vi "获取公式.vi"(10 "量程选择":enum16{"低量程", "高量程", "0-2量程"}(ring), 11 "测量模式(公式)":u16(ring)=1 items=["水样测试"=1, "标样核查"=2, "零点核查"=3, "跨度核查"=4, "空白测试"=5, "平行样"=6, "加标回收"=7]) -> (3 "方程系数":cluster{"K":dbl, "b":dbl, "X^2":dbl} {"X^2" format="%#.6g"; "b" format="%#.6g"; "K" format="%#.6g"})   [LabVIEW 2016, in "斯坦道CODMn.lvlib"]
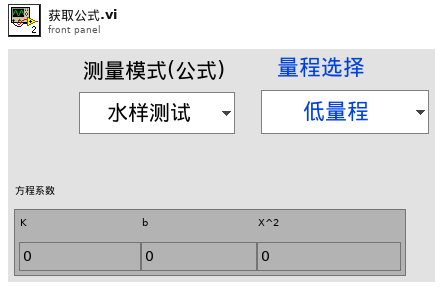
[diagram p1: front panel]
types:
  T1 = cluster{"数组 2[0]":sgl, "数组 2[1]":sgl, "数组 2[2]":sgl, "数组 2[3]":sgl, "数组 2[4]":sgl, "数组 2[5]":sgl, "数组 2[6]":sgl, "数组 2[7]":sgl, "数组 2[8]":sgl, "数组 2[9]":sgl, "数组 2[10]":sgl, "数组 2[11]":sgl, "数组 2[12]":sgl, "数组 2[13]":sgl, "数组 2[14]":sgl, "数组 2[15]":sgl, "数组 2[16]":sgl, "数组 2[17]":sgl, "数组 2[18]":sgl, "数组 2[19]":sgl, "数组 2[20]":sgl, "数组 2[21]":sgl, "数组 2[22]":sgl, "数组 2[23]":sgl, "数组 2[24]":sgl, "数组 2[25]":sgl, "数组 2[26]":sgl, "数组 2[27]":sgl, "数组 2[28]":sgl, "数组 2[29]":sgl, "数组 2[30]":sgl, "数组 2[31]":sgl, "数组 2[32]":sgl, "数组 2[33]":sgl, "数组 2[34]":sgl, "数组 2[35]":sgl, "数组 2[36]":sgl, "数组 2[37]":sgl, "数组 2[38]":sgl, "数组 2[39]":sgl, "数组 2[40]":sgl, "数组 2[41]":sgl}
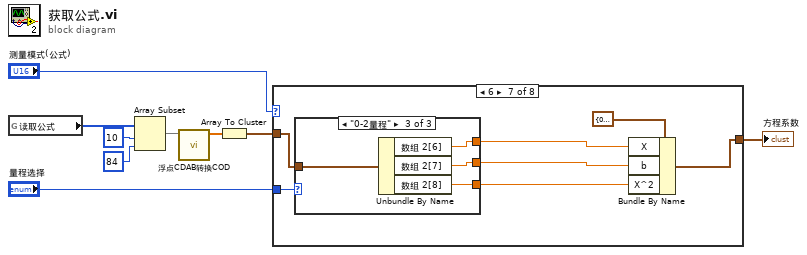
[diagram p0: block diagram]
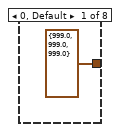
[diagram p2: hidden frame]
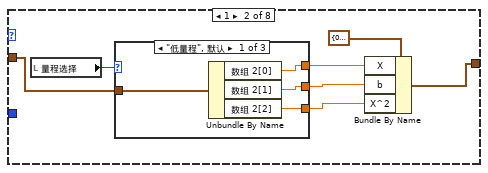
[diagram p3: hidden frame]
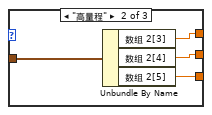
[diagram p4: hidden frame]
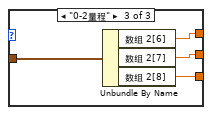
[diagram p5: hidden frame]
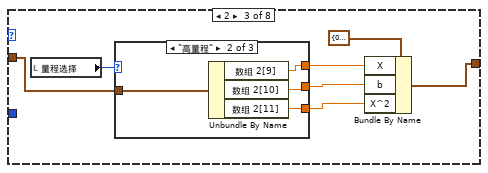
[diagram p6: hidden frame]
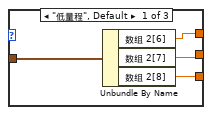
[diagram p7: hidden frame]
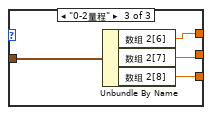
[diagram p8: hidden frame]
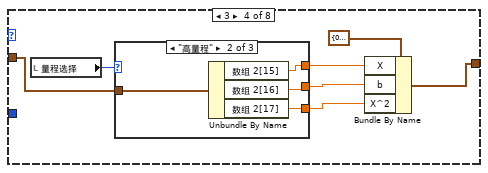
[diagram p9: hidden frame]
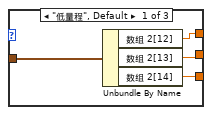
[diagram p10: hidden frame]
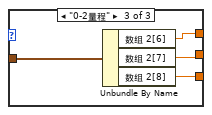
[diagram p11: hidden frame]
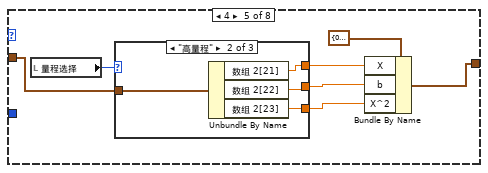
[diagram p12: hidden frame]
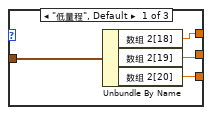
[diagram p13: hidden frame]
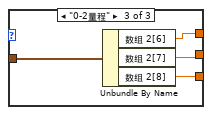
[diagram p14: hidden frame]
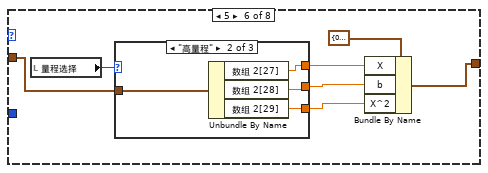
[diagram p15: hidden frame]
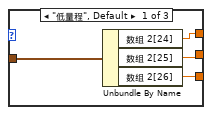
[diagram p16: hidden frame]
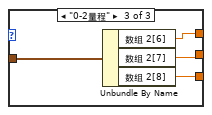
[diagram p17: hidden frame]
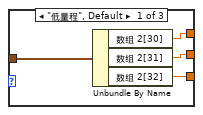
[diagram p18: hidden frame]
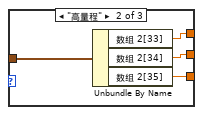
[diagram p19: hidden frame]
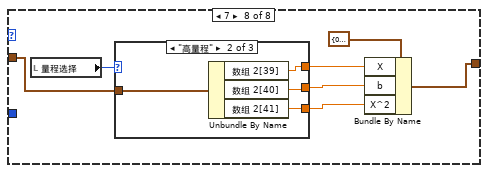
[diagram p20: hidden frame]
diagram:
  n1 = global read "COD内部交互全局.vi" "读取公式"() -> (w9:u16[])
  n2 = Array Subset(array=w9, index=10 ("索引"), length=84 ("长度")) -> (w6:u16[])
  n3 = call "浮点CDAB转换COD.vi"("数组"=w6) -> ("数组 2"=w7:sgl[])  [unwired: 10 in]
  n4 = Array To Cluster(array=w7) -> (cluster=w8:T1)
  n5 = case shown="6" "测量模式(公式)" {
    tunnel: [cluster{"X":dbl, "b":dbl, "X^2":dbl} {"X"=999.0, "b"=999.0, "X^2"=999.0} ("方程系数") w12 w31 w50 w69 w88 w108 w126] -> w1
    tunnel: w8 -> [_ w11 w30 w49 w68 w87 w107 w125]
    tunnel: "量程选择" -> [_ _ _ _ _ _ w106 _]
    frame 0, Default {
    }
    frame 1 {
      n6 = local read "量程选择"() -> (w14:enum16{"低量程", "高量程", "0-2量程"})
      n7 = case shown="\"低量程\", 默认" w14 {
        tunnel: w11 -> [w21 w25 w29]
        tunnel: [w20 w24 w28] -> w17
        tunnel: [w19 w23 w27] -> w16
        tunnel: [w18 w22 w26] -> w15
        frame "低量程", Default {
          n8 = Unbundle By Name(w21) -> ("数组 2[0]"=w20:sgl, "数组 2[1]"=w19:sgl, "数组 2[2]"=w18:sgl)
        }
        frame "高量程" {
          n9 = Unbundle By Name(w25) -> ("数组 2[3]"=w24:sgl, "数组 2[4]"=w23:sgl, "数组 2[5]"=w22:sgl)
        }
        frame "0-2量程" {
          n10 = Unbundle By Name(w29) -> ("数组 2[6]"=w28:sgl, "数组 2[7]"=w27:sgl, "数组 2[8]"=w26:sgl)
        }
      }
      n11 = Bundle By Name(cluster=cluster{"X":dbl, "b":dbl, "X^2":dbl} {"X"=0.0, "b"=0.0, "X^2"=0.0} ("方程系数"), "X"=w17, "b"=w16, "X^2"=w15) -> (w12:cluster{"X":dbl, "b":dbl, "X^2":dbl})
    }
    frame 2 {
      n12 = local read "量程选择"() -> (w33:enum16{"低量程", "高量程", "0-2量程"})
      n13 = case shown="\"高量程\"" w33 {
        tunnel: w30 -> [w40 w44 w48]
        tunnel: [w39 w43 w47] -> w36
        tunnel: [w38 w42 w46] -> w35
        tunnel: [w37 w41 w45] -> w34
        frame "低量程", Default {
          n14 = Unbundle By Name(w40) -> ("数组 2[6]"=w39:sgl, "数组 2[7]"=w38:sgl, "数组 2[8]"=w37:sgl)
        }
        frame "高量程" {
          n15 = Unbundle By Name(w44) -> ("数组 2[9]"=w43:sgl, "数组 2[10]"=w42:sgl, "数组 2[11]"=w41:sgl)
        }
        frame "0-2量程" {
          n16 = Unbundle By Name(w48) -> ("数组 2[6]"=w47:sgl, "数组 2[7]"=w46:sgl, "数组 2[8]"=w45:sgl)
        }
      }
      n17 = Bundle By Name(cluster=cluster{"X":dbl, "b":dbl, "X^2":dbl} {"X"=0.0, "b"=0.0, "X^2"=0.0} ("方程系数"), "X"=w36, "b"=w35, "X^2"=w34) -> (w31:cluster{"X":dbl, "b":dbl, "X^2":dbl})
    }
    frame 3 {
      n18 = local read "量程选择"() -> (w52:enum16{"低量程", "高量程", "0-2量程"})
      n19 = case shown="\"高量程\"" w52 {
        tunnel: w49 -> [w59 w63 w67]
        tunnel: [w58 w62 w66] -> w55
        tunnel: [w57 w61 w65] -> w54
        tunnel: [w56 w60 w64] -> w53
        frame "低量程", Default {
          n20 = Unbundle By Name(w59) -> ("数组 2[12]"=w58:sgl, "数组 2[13]"=w57:sgl, "数组 2[14]"=w56:sgl)
        }
        frame "高量程" {
          n21 = Unbundle By Name(w63) -> ("数组 2[15]"=w62:sgl, "数组 2[16]"=w61:sgl, "数组 2[17]"=w60:sgl)
        }
        frame "0-2量程" {
          n22 = Unbundle By Name(w67) -> ("数组 2[6]"=w66:sgl, "数组 2[7]"=w65:sgl, "数组 2[8]"=w64:sgl)
        }
      }
      n23 = Bundle By Name(cluster=cluster{"X":dbl, "b":dbl, "X^2":dbl} {"X"=0.0, "b"=0.0, "X^2"=0.0} ("方程系数"), "X"=w55, "b"=w54, "X^2"=w53) -> (w50:cluster{"X":dbl, "b":dbl, "X^2":dbl})
    }
    frame 4 {
      n24 = local read "量程选择"() -> (w71:enum16{"低量程", "高量程", "0-2量程"})
      n25 = case shown="\"高量程\"" w71 {
        tunnel: w68 -> [w78 w82 w86]
        tunnel: [w77 w81 w85] -> w74
        tunnel: [w76 w80 w84] -> w73
        tunnel: [w75 w79 w83] -> w72
        frame "低量程", Default {
          n26 = Unbundle By Name(w78) -> ("数组 2[18]"=w77:sgl, "数组 2[19]"=w76:sgl, "数组 2[20]"=w75:sgl)
        }
        frame "高量程" {
          n27 = Unbundle By Name(w82) -> ("数组 2[21]"=w81:sgl, "数组 2[22]"=w80:sgl, "数组 2[23]"=w79:sgl)
        }
        frame "0-2量程" {
          n28 = Unbundle By Name(w86) -> ("数组 2[6]"=w85:sgl, "数组 2[7]"=w84:sgl, "数组 2[8]"=w83:sgl)
        }
      }
      n29 = Bundle By Name(cluster=cluster{"X":dbl, "b":dbl, "X^2":dbl} {"X"=0.0, "b"=0.0, "X^2"=0.0} ("方程系数"), "X"=w74, "b"=w73, "X^2"=w72) -> (w69:cluster{"X":dbl, "b":dbl, "X^2":dbl})
    }
    frame 5 {
      n30 = local read "量程选择"() -> (w90:enum16{"低量程", "高量程", "0-2量程"})
      n31 = case shown="\"高量程\"" w90 {
        tunnel: w87 -> [w97 w101 w105]
        tunnel: [w96 w100 w104] -> w93
        tunnel: [w95 w99 w103] -> w92
        tunnel: [w94 w98 w102] -> w91
        frame "低量程", Default {
          n32 = Unbundle By Name(w97) -> ("数组 2[24]"=w96:sgl, "数组 2[25]"=w95:sgl, "数组 2[26]"=w94:sgl)
        }
        frame "高量程" {
          n33 = Unbundle By Name(w101) -> ("数组 2[27]"=w100:sgl, "数组 2[28]"=w99:sgl, "数组 2[29]"=w98:sgl)
        }
        frame "0-2量程" {
          n34 = Unbundle By Name(w105) -> ("数组 2[6]"=w104:sgl, "数组 2[7]"=w103:sgl, "数组 2[8]"=w102:sgl)
        }
      }
      n35 = Bundle By Name(cluster=cluster{"X":dbl, "b":dbl, "X^2":dbl} {"X"=0.0, "b"=0.0, "X^2"=0.0} ("方程系数"), "X"=w93, "b"=w92, "X^2"=w91) -> (w88:cluster{"X":dbl, "b":dbl, "X^2":dbl})
    }
    frame 6 {
      n36 = case shown="\"0-2量程\"" w106 {
        tunnel: w107 -> [w116 w120 w124]
        tunnel: [w115 w119 w123] -> w112
        tunnel: [w114 w118 w122] -> w111
        tunnel: [w113 w117 w121] -> w110
        frame "低量程", Default {
          n37 = Unbundle By Name(w116) -> ("数组 2[30]"=w115:sgl, "数组 2[31]"=w114:sgl, "数组 2[32]"=w113:sgl)
        }
        frame "高量程" {
          n38 = Unbundle By Name(w120) -> ("数组 2[33]"=w119:sgl, "数组 2[34]"=w118:sgl, "数组 2[35]"=w117:sgl)
        }
        frame "0-2量程" {
          n39 = Unbundle By Name(w124) -> ("数组 2[6]"=w123:sgl, "数组 2[7]"=w122:sgl, "数组 2[8]"=w121:sgl)
        }
      }
      n40 = Bundle By Name(cluster=cluster{"X":dbl, "b":dbl, "X^2":dbl} {"X"=0.0, "b"=0.0, "X^2"=0.0} ("方程系数"), "X"=w112, "b"=w111, "X^2"=w110) -> (w108:cluster{"X":dbl, "b":dbl, "X^2":dbl})
    }
    frame 7 {
      n41 = local read "量程选择"() -> (w128:enum16{"低量程", "高量程", "0-2量程"})
      n42 = case shown="\"高量程\"" w128 {
        tunnel: w125 -> [w135 w139 w143]
        tunnel: [w134 w138 w142] -> w131
        tunnel: [w133 w137 w141] -> w130
        tunnel: [w132 w136 w140] -> w129
        frame "低量程", Default {
          n43 = Unbundle By Name(w135) -> ("数组 2[36]"=w134:sgl, "数组 2[37]"=w133:sgl, "数组 2[38]"=w132:sgl)
        }
        frame "高量程" {
          n44 = Unbundle By Name(w139) -> ("数组 2[39]"=w138:sgl, "数组 2[40]"=w137:sgl, "数组 2[41]"=w136:sgl)
        }
        frame "0-2量程" {
          n45 = Unbundle By Name(w143) -> ("数组 2[6]"=w142:sgl, "数组 2[7]"=w141:sgl, "数组 2[8]"=w140:sgl)
        }
      }
      n46 = Bundle By Name(cluster=cluster{"X":dbl, "b":dbl, "X^2":dbl} {"X"=0.0, "b"=0.0, "X^2"=0.0} ("方程系数"), "X"=w131, "b"=w130, "X^2"=w129) -> (w126:cluster{"X":dbl, "b":dbl, "X^2":dbl})
    }
  }
  "方程系数" <- w1
